vi "Check-Corrected-image-storage.vi"(8 "error in":errorcluster, 10 "Correct. params. ref.":refnum<data-value>, 11 "Save?":bool) -> (0 "error IO":errorcluster, 3 "Passed?":bool)   [LabVIEW 2013, in "CameraVision.lvlib" / "CV-Storage.lvclass"]
uses:
  CV-Storage.lvclass
  Correction/CV-Correction.lvclass
  Correction/CV-Correction.lvclass/CV-Correction.ctl
  Correction/Read Background correction.vi
  Correction/Read Hotpixel correction.vi
  Correction/Read Image smoothing.vi
  Correction/Read 2nd image correlation.vi
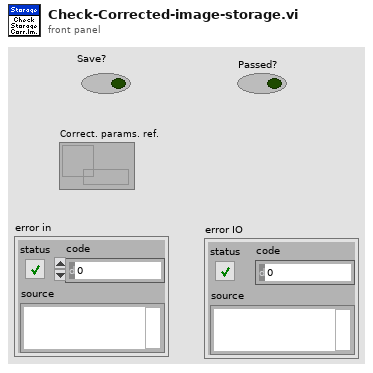
[diagram p1: front panel]
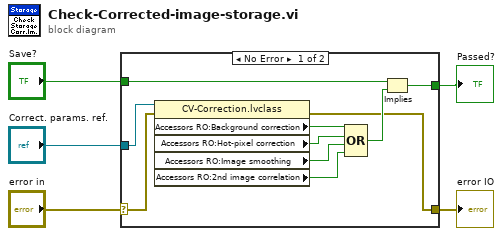
[diagram p0: block diagram]
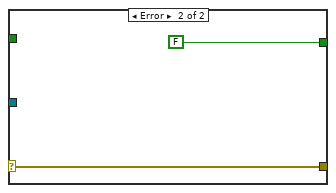
[diagram p2: hidden frame]
diagram:
  n1 = case shown="No Error" "error in" {
    selector: "error in" -> [w7 w16]
    tunnel: "Correct. params. ref." -> [w12 _]
    tunnel: [w6 w16] -> w4
    tunnel: [w14 FALSE] -> w5
    tunnel: "Save?" -> [w13 _]
    frame No Error {
      n2 = property class="CV-Correction.lvclass"(reference=w12, error in=w7) -> (error out=w6:errorcluster, "Accessors RO:Background correction"=w11:bool, "Accessors RO:Hot-pixel correction"=w10:bool, "Accessors RO:Image smoothing"=w9:bool, "Accessors RO:2nd image correlation"=w8:bool)  [unwired: 1 out]
      n3 = Compound Arithmetic op=OR(w11, w10, w9, w8) -> (w15:bool)
      n4 = Implies(1:w15, 2:w13) -> (0:w14:bool)
    }
    frame Error {
    }
  }
  "Passed?" <- w5
  "error IO" <- w4
